vi "DB Get Defects from pure ID.vi"(6 "Ignore Incomplete":bool, 8 "error in (no error)":errorcluster, 9 "Ignore Location":bool, 10 "Defect Free Structure ID":string, 11 "connection reference in":T2) -> (0 "error out":errorcluster, 1 "String Data":string[][](array[string]), 2 "Defects Array":T1(array[cluster]), 3 "connection reference out":T2)   [LabVIEW 2010]
uses:
  <vilib>/addons/database/Connection.llb/Conn ObjectReference.ctl
  <vilib>/addons/database/_DB Variant To Data/Database Variant To Data.xnode
  <vilib>/addons/database/Connection.llb/Conn Execute.vi
  <vilib>/addons/database/Recordset.llb/Rec Fetch Recordset Data (R).vi
  <vilib>/addons/database/Recordset.llb/Rec Destroy - Connection.vi
  <vilib>/addons/database/NI_Database_API.lvlib
panel:
  out "concatenated string":string
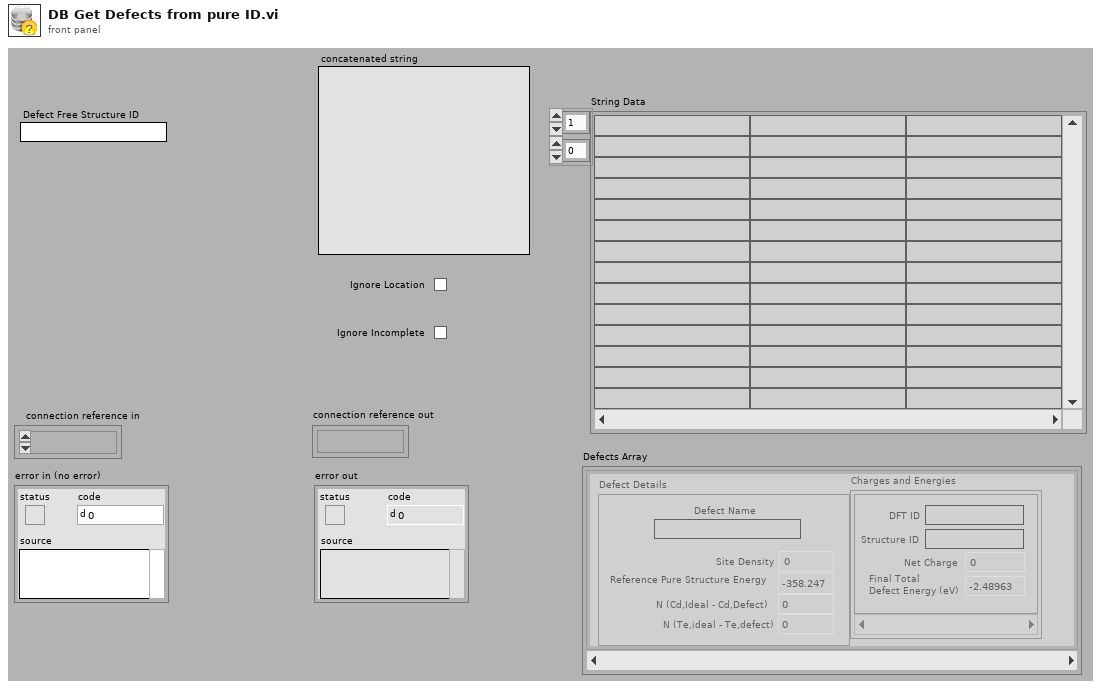
[diagram p1: front panel]
types:
  T1 = cluster{"Defect Details":cluster{"Defect Name":string, "Site Density":dbl, "Reference Pure Structure Energy":dbl, "N (Cd,Ideal - Cd,Defect)":i32, "N (Te,ideal - Te,defect)":i32}, "Charges and Energies":cluster{"DFT ID":string, "Structure ID":string, "Net Charge":i32, "Final Total \nDefect Energy (eV)":dbl}[]}[]
  T2 = typedef "NI_Database_API.lvlib/Conn ObjectReference.ctl" = refnum<k1>
  T3 = typedef "NI_Database_API.lvlib/Rec ObjectReference.ctl" = refnum<k1>
  T4 = cluster{"data":string, "data":string, i32, dbl}[]
  T5 = cluster{cluster{"data":string, dbl, dbl, i32, i32}, cluster{"data":string, "data":string, i32, dbl}[]}
  T6 = cluster{"Defect Details":cluster{"data":string, "Site Density":dbl, "Reference Pure Structure Energy":dbl, "N (Cd,Ideal - Cd,Defect)":i32, "N (Te,ideal - Te,defect)":i32}, "Charges and Energies":cluster{"data":string, "data":string, "Net Charge":i32, "Final Total \nDefect Energy (eV)":dbl}[]}[]
  T7 = cluster{"Defect Details":cluster{"Defect Name":string, "Site Density":dbl, "Reference Pure Structure Energy":dbl, "N (Cd,Ideal - Cd,Defect)":i32, "N (Te,ideal - Te,defect)":i32}, "Charges and Energies":cluster{"DFT ID":string, "Structure ID":string, "Net Charge":i32, "Final Total \nDefect Energy (eV)":dbl}[]}
  T8 = cluster{"DFT ID":string, "Structure ID":string, "Net Charge":i32, "Final Total \nDefect Energy (eV)":dbl}[]
  T9 = cluster{"data":string, "data":string, "Net Charge":i32, "Final Total \nDefect Energy (eV)":dbl}[]
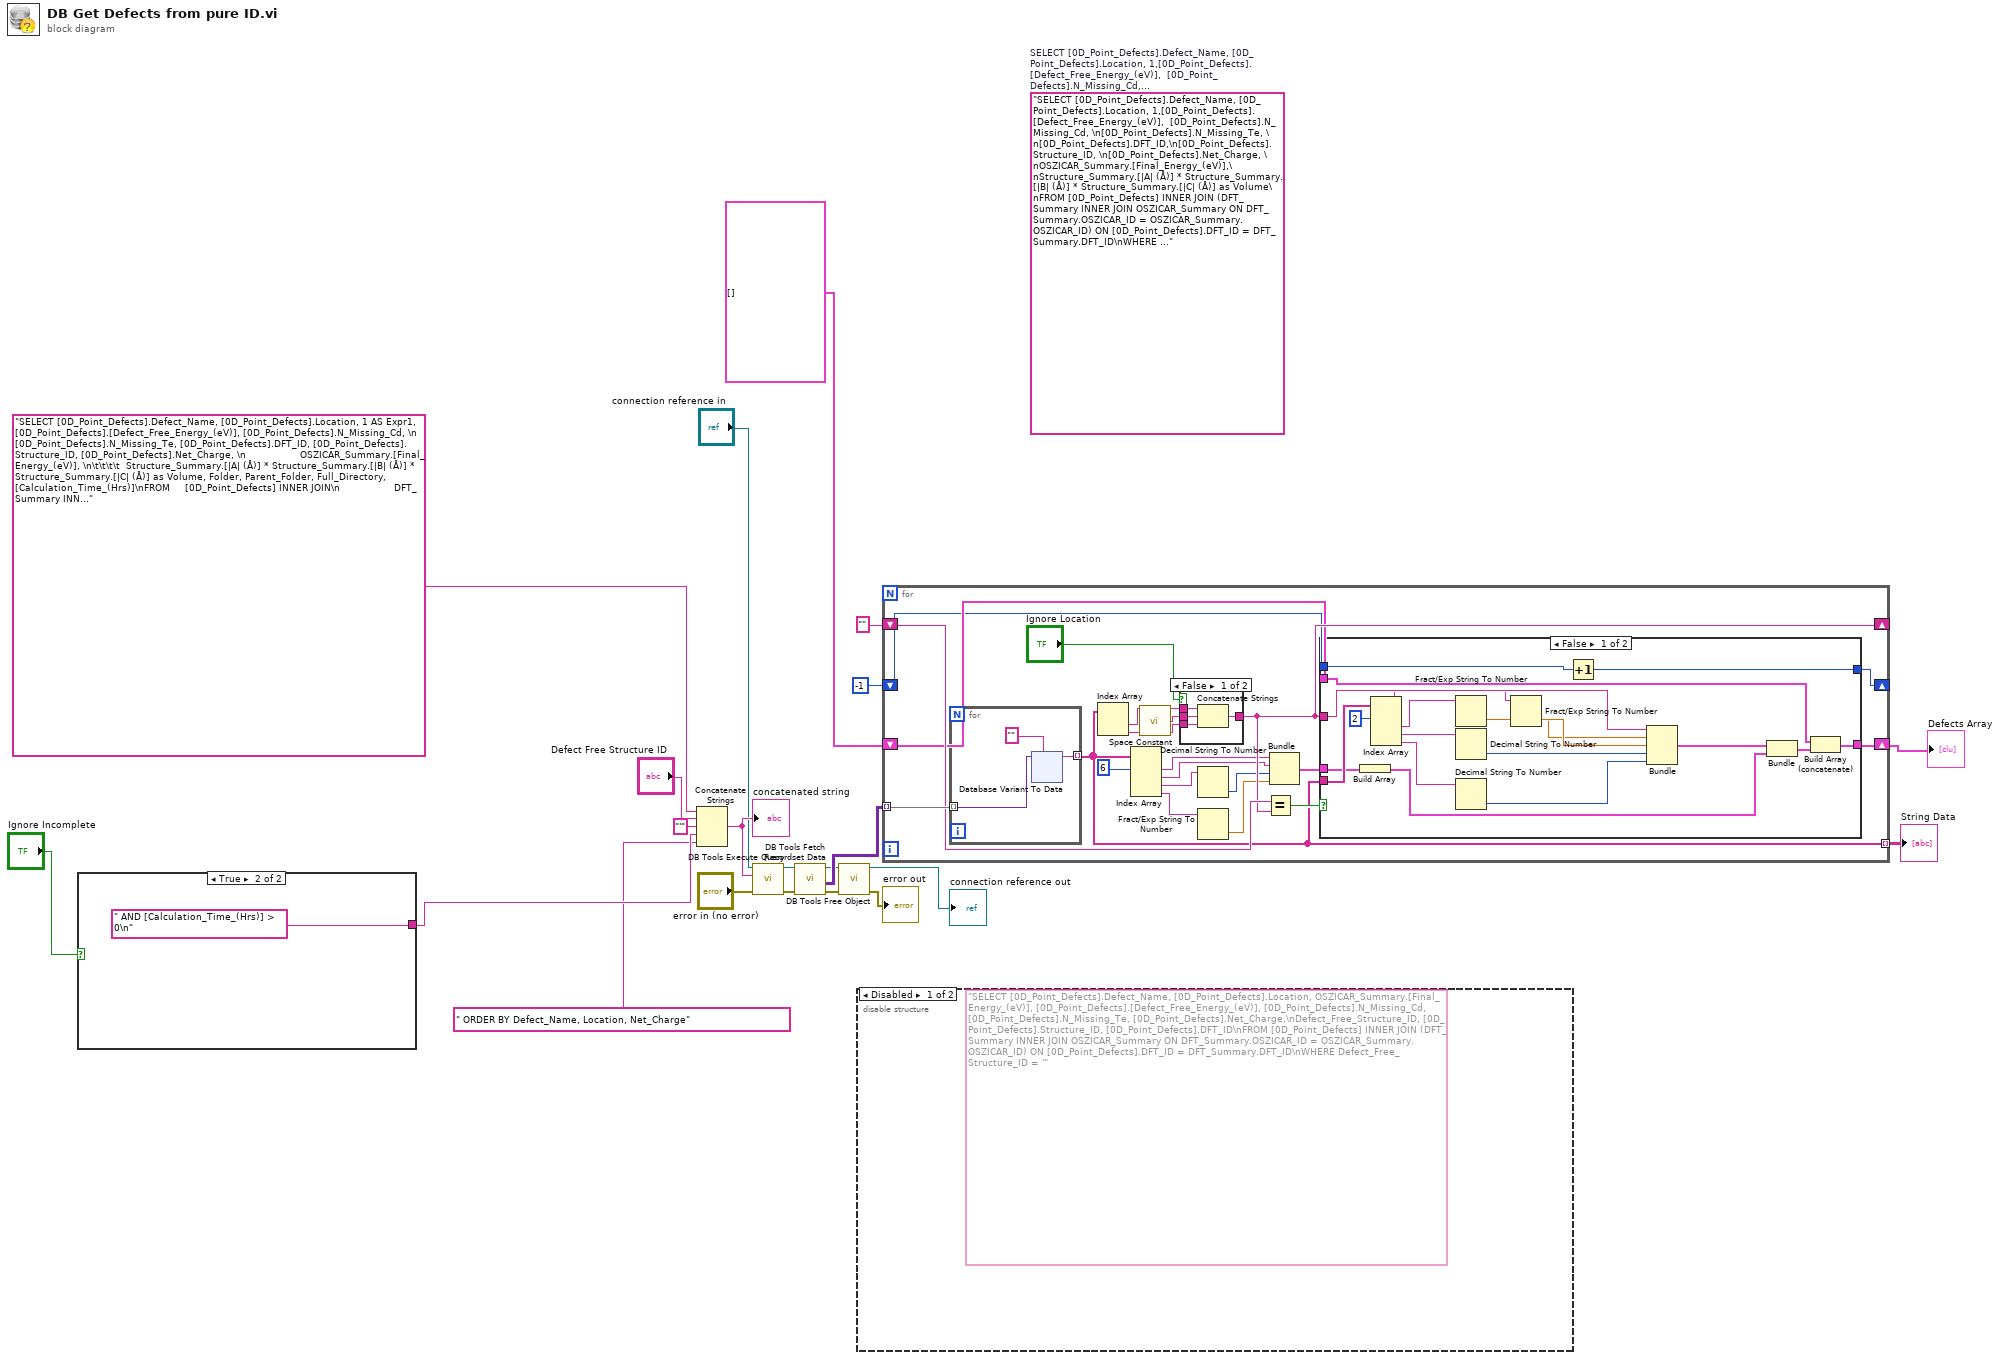
[diagram p0: block diagram]
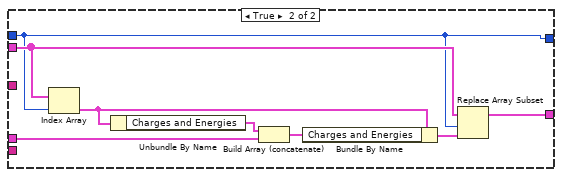
[diagram p5: hidden frame]
diagram:
  (unwired) "SELECT [0D_Point_Defects].Defect_Name, [0D_Point_Defects].Location, 1,[0D_Point_Defects].[Defect_Free_Energy_(eV)],  [0D_Point_Defects].N_Missing_Cd, \n[0D_Point_Defects].N_Missing_Te, \n[0D_Point_Defects].DFT_ID,\n[0D_Point_Defects].Structure_ID, \n[0D_Point_Defects].Net_Charge, \nOSZICAR_Summary.[Final_Energy_(eV)],\nStructure_Summary.[|A| (Å)] * Structure_Summary.[|B| (Å)] * Structure_Summary.[|C| (Å)] as Volume\nFROM [0D_Point_Defects] INNER JOIN (DFT_Summary INNER JOIN OSZICAR_Summary ON DFT_Summary.OSZICAR_ID = OSZICAR_Summary.OSZICAR_ID) ON [0D_Point_Defects].DFT_ID = DFT_Summary.DFT_ID\nWHERE Defect_Free_Structure_ID = '"  # SELECT [0D_Point_Defects].Defect_Name, [0D_Point_Defects].Location, 1,[0D_Point_Defects].[Defect_Free_Energy_(eV)],  [0D_Point_Defects].N_Missing_Cd,  [0D_Point_Defects].N_Missing_Te,  [0D_Point_Defects].DFT_ID, [0D_Point_Defects].Structure_ID,  [0D_Point_Defects].Net_Charge,  OSZICAR_Summary.[Final_Energy_(eV)], Structure_Summary.[|A| (Å)] * Structure_Summary.[|B| (Å)] * Structure_Summary.[|C| (Å)] as Volume FROM [0D_Point_Defects] INNER JOIN (DFT_Summary INNER JOIN OSZICAR_Summary ON DFT_Summary.OSZICAR_ID = OSZICAR_Summary.OSZICAR_ID) ON [0D_Point_Defects].DFT_ID = DFT_Summary.DFT_ID WHERE Defect_Free_Structure_ID = '
  n1 = case shown="True" "Ignore Incomplete" {
    tunnel: [_ " AND [Calculation_Time_(Hrs)] > 0\n" ("string")] -> w2
    frame False {
    }
    frame True {
    }
  }
  n2 = Concatenate Strings("SELECT [0D_Point_Defects].Defect_Name, [0D_Point_Defects].Location, 1 AS Expr1, [0D_Point_Defects].[Defect_Free_Energy_(eV)], [0D_Point_Defects].N_Missing_Cd, \n                  [0D_Point_Defects].N_Missing_Te, [0D_Point_Defects].DFT_ID, [0D_Point_Defects].Structure_ID, [0D_Point_Defects].Net_Charge, \n                  OSZICAR_Summary.[Final_Energy_(eV)], \n\t\t\t\t  Structure_Summary.[|A| (Å)] * Structure_Summary.[|B| (Å)] * Structure_Summary.[|C| (Å)] as Volume, Folder, Parent_Folder, Full_Directory, [Calculation_Time_(Hrs)]\nFROM     [0D_Point_Defects] INNER JOIN\n                  DFT_Summary INNER JOIN\n                  OSZICAR_Summary ON DFT_Summary.OSZICAR_ID = OSZICAR_Summary.OSZICAR_ID ON [0D_Point_Defects].DFT_ID = DFT_Summary.DFT_ID INNER JOIN\n                  Structure_Summary ON [0D_Point_Defects].Structure_ID = Structure_Summary.Structure_ID\nWHERE  [0D_Point_Defects].Defect_Free_Structure_ID = '", "Defect Free Structure ID", "'" ("string"), w2, " ORDER BY Defect_Name, Location, Net_Charge") -> (w15:string)
  "concatenated string" <- w15
  n3 = call-poly <vilib>:"DB Tools Execute Query.vi"("error in (no error)"="error in (no error)", "SQL query"=w15, "connection reference"="connection reference in") -> ("error out"=w13:errorcluster, "recordset reference"=w14:T3)  [unwired: 5 in]
  n4 = call-poly <vilib>:"DB Tools Fetch Recordset Data.vi"("error in (no error)"=w13, "recordset reference"=w14) -> ("error out"=w18:errorcluster, "recordset data"=w21:variant[][], "recordset reference out"=w17:T3)  [unwired: 3 in]
  n5 = call-poly <vilib>:"DB Tools Free Object.vi"("error in (no error)"=w18, "recordset reference"=w17) -> ("error out"=→"error out":errorcluster, "connection reference"=→"connection reference out":T2)  [unwired: 8 in]
  n6 = disable-structure shown="Disabled" {
    frame Disabled {
      (unwired) "SELECT [0D_Point_Defects].Defect_Name, [0D_Point_Defects].Location, OSZICAR_Summary.[Final_Energy_(eV)], [0D_Point_Defects].[Defect_Free_Energy_(eV)], [0D_Point_Defects].N_Missing_Cd, [0D_Point_Defects].N_Missing_Te, [0D_Point_Defects].Net_Charge,\nDefect_Free_Structure_ID, [0D_Point_Defects].Structure_ID, [0D_Point_Defects].DFT_ID\nFROM [0D_Point_Defects] INNER JOIN (DFT_Summary INNER JOIN OSZICAR_Summary ON DFT_Summary.OSZICAR_ID = OSZICAR_Summary.OSZICAR_ID) ON [0D_Point_Defects].DFT_ID = DFT_Summary.DFT_ID\nWHERE Defect_Free_Structure_ID = '"
    }
    frame Enabled {
    }
  }
  n7 = for {
    tunnel: w21 -> [w43] mode=indexing
    shift-right: [w37] -> _
    shift-left: "" -> [w42]
    shift-right: [w36] -> w5
    shift-left: T1 [] ("Defects Array 2") -> [w35]
    shift-right: [w33] -> _
    shift-left: -1 -> [w34]
    tunnel: [w32] -> w7 mode=indexing
    n8 = for {
      tunnel: w43 -> [w78] mode=indexing
      tunnel: [w76] -> w32 mode=indexing
      n9 = xnode "Database Variant To Data"("database variant"=w78, "type"="") -> ("data"=w76:string)  [unwired: 1 in, 1 out]
    }
    n10 = Index Array(array=w32) -> (element #1=w40:string, element #2=w38:string)  [unwired: 2 in]
    n11 = Index Array(array=w32, index #1=6 ("index")) -> (element #1=w30:string, element #2=w29:string, element #3=w25:string, element #4=w24:string)  [unwired: 3 in]
    n12 = call <vilib>:"Space Constant.vi"() -> ("String"=w39:string)
    n13 = case shown="False" "Ignore Location" {
      tunnel: w40 -> [w47 w48]
      tunnel: w39 -> [w46 _]
      tunnel: w38 -> [w45 _]
      tunnel: [w44 w48] -> w37
      frame False {
        n14 = Concatenate Strings(w47, w46, w45) -> (w44:string)
      }
      frame True {
      }
    }
    n15 = Decimal String To Number(string=w25) -> (number=w28:i32)  [unwired: 2 in, 1 out]
    n16 = Fract/Exp String To Number(string=w24) -> (number=w27:dbl)  [unwired: 3 in, 1 out]
    n17 = Equal?(x=w42, y=w37) -> (x = y?=w41:bool)
    n18 = Bundle("data"=w30, "data"=w29, w28, w27) -> (w26:cluster{"data":string, "data":string, i32, dbl})  [unwired: 1 in]
    n19 = case shown="False" w41 {
      tunnel: w32 -> [w67 _]
      tunnel: w37 -> [w66 _]
      tunnel: [w56 w74] -> w36
      tunnel: w35 -> [w55 w73]
      tunnel: w34 -> [w54 w69]
      tunnel: [w53 w69] -> w33
      tunnel: w26 -> [w52 w68]
      frame False {
        n20 = Build Array(w52) -> (w58:T4)
        n21 = Index Array(array=w67, index #1=2 ("index")) -> (element #1=w50:string, element #2=w65:string, element #3=w63:string, element #4=w61:string)  [unwired: 3 in]
        n22 = Fract/Exp String To Number(string=w65) -> (number=w64:dbl)  [unwired: 3 in, 1 out]
        n23 = Decimal String To Number(string=w63) -> (number=w62:i32)  [unwired: 2 in, 1 out]
        n24 = Decimal String To Number(string=w61) -> (number=w60:i32)  [unwired: 2 in, 1 out]
        n25 = Fract/Exp String To Number(string=w50) -> (number=w49:dbl)  [unwired: 3 in, 1 out]
        n26 = Increment(x=w54) -> (x+1=w53:i32)
        n27 = Bundle("data"=w66, w49, w64, w62, w60) -> (w59:cluster{"data":string, dbl, dbl, i32, i32})  [unwired: 1 in]
        n28 = Bundle(w59, w58) -> (w57:T5)  [unwired: 1 in]
        n29 = Build Array (concatenate)(w55, w57) -> (w56:T6)
      }
      frame True {
        n30 = Index Array(array=w73, index=w69) -> (element=w71:T7)
        n31 = Unbundle By Name(w71) -> ("Charges and Energies"=w72:T8)
        n32 = Build Array (concatenate)(w72, w68) -> (w75:T9)
        n33 = Bundle By Name(cluster=w71, "Charges and Energies"=w75) -> (w70:T7)
        n34 = Replace Array Subset(array=w73, new element=w70, index=w69) -> (w74:T1)
      }
    }
  }
  "String Data" <- w7
  "Defects Array" <- w5
